vi "Read BIO.vi"(8 "error in (no error)":errorcluster, 11 "SSL Socket in":refnum<class "SSL Socket.lvclass">) -> (0 "error out":errorcluster, 2 "SSL_Lib.lvlib:BIO.lvclass":refnum<class "BIO.lvclass">, 3 "SSL Socket out":refnum<class "SSL Socket.lvclass">)   [LabVIEW 2013, in "OpenSSL Socket.lvlib" / "SSL Socket.lvclass"]
uses:
  SSL Socket.lvclass
  SSL_Lib/BIO/BIO.lvclass
  SSL Socket.lvclass/SSL Socket.ctl
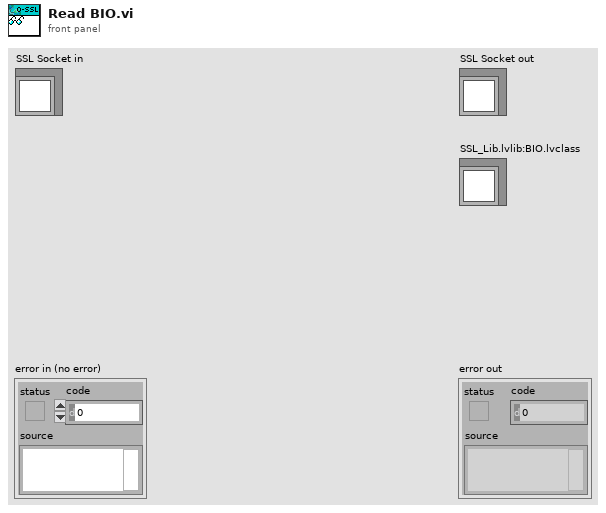
[diagram p1: front panel]
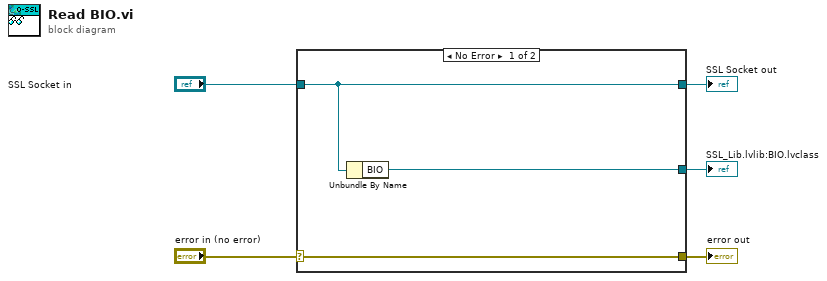
[diagram p0: block diagram]
diagram:
  n1 = case shown="No Error" "error in (no error)" {
    selector: "error in (no error)" -> [w8 w9]
    tunnel: [w8 w9] -> w4
    tunnel: [w7 w10] -> w2
    tunnel: "SSL Socket in" -> [w7 w10]
    tunnel: [w6 _] -> w1
    frame No Error {
      n2 = Unbundle By Name(w7) -> ("BIO"=w6:refnum<class "BIO.lvclass">)
    }
    frame Error {
    }
  }
  "error out" <- w4
  "SSL Socket out" <- w2
  "SSL_Lib.lvlib:BIO.lvclass" <- w1
